vi "check validity of conjugate complex.vi"(8 "tolerance for complex pair":dbl=1e-10, 9 "min distance to (z)*":dbl, 10 "min distance index":i32, 11 "Complex Numbers":cdb[](array[numeric])) -> (3 "out of tolerance?":bool)   [LabVIEW 2020, in "NI_AALPro.lvlib"]
uses:
  NI_AALPro.lvlib
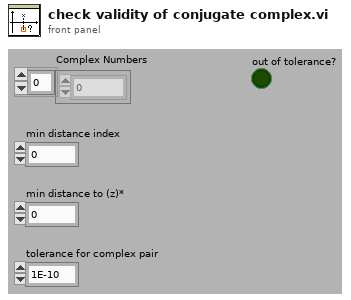
[diagram p1: front panel]
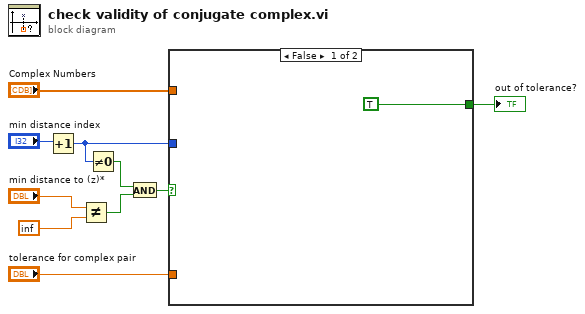
[diagram p0: block diagram]
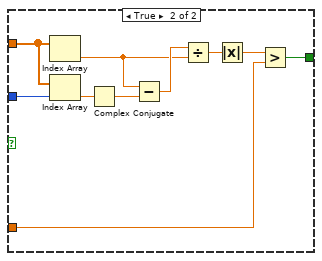
[diagram p2: hidden frame]
diagram:
  n1 = Increment(x="min distance index") -> (x+1=w4:i32)
  n2 = Not Equal?(x="min distance to (z)*", y=inf) -> (x != y?=w3:bool)
  n3 = Not Equal To 0?(x=w4) -> (x != 0?=w2:bool)
  n4 = And(x=w2, y=w3) -> (x .and. y?=w1:bool)
  n5 = case shown="False" w1 {
    tunnel: "Complex Numbers" -> [_ w20]
    tunnel: w4 -> [_ w21]
    tunnel: "tolerance for complex pair" -> [_ w13]
    tunnel: [TRUE w12] -> w5
    frame False {
    }
    frame True {
      n6 = Index Array(array=w20) -> (element=w16:cdb)  [unwired: 1 in]
      n7 = Index Array(array=w20, index=w21) -> (element=w19:cdb)
      n8 = Complex Conjugate(1:w19) -> (0:w18:cdb)
      n9 = Subtract(x=w16, y=w18) -> (x-y=w17:cdb)
      n10 = Divide(x=w17, y=w16) -> (x/y=w15:cdb)
      n11 = Absolute Value(x=w15) -> (abs(x)=w14:dbl)
      n12 = Greater?(x=w14, y=w13) -> (0:w12:bool)
    }
  }
  "out of tolerance?" <- w5
